vi "lvlib To class File Path.vi"(10 "lvlib File Path":path) -> (2 "class File Path":path)   [LabVIEW 2021, in "_Shared.lvlib"]
uses:
  _Rename/_Rename/_Rename.lvclass/_Rename.ctl
  _Shared.lvlib
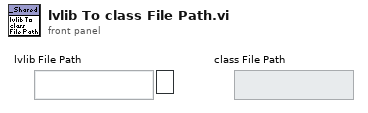
[diagram p1: front panel]
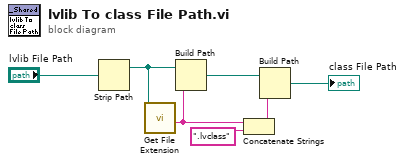
[diagram p0: block diagram]
diagram:
  n1 = Strip Path(path="lvlib File Path") -> (stripped path=w4:path)  [unwired: 1 out]
  n2 = call <vilib>:"Get File Extension.vi"("file"=w4) -> ("filename without extension"=w1:string)  [unwired: 6 in, 4 out]
  n3 = Build Path(base path=w4, name or relative path=w1) -> (appended path=w3:path)
  n4 = Concatenate Strings(w1, ".lvclass" ("string")) -> (w7:string)
  n5 = Build Path(base path=w3, name or relative path=w7) -> (appended path=→"class File Path":path)
